vi "Read Camera Status 2.vi"(8 "error in (no error)":errorcluster, 11 "Interface in":refnum<class "Interface.lvclass">) -> (0 "error out":errorcluster, 2 "Camera Status":T1={"CUBE_EXPOSURE_TIME"=0.0, "CUBES_DONE"=1, "LAST_IMAGE_NAME"="", "DISK_SPACE"=0, "FRAMES_DONE"=0, "CCD_STATUS"="", "CURRENT_TEMPERATURE"=0, "TEMPERATURE_STATUS"="", "FRAME_EXPOSURE_TIME"=0, "CCD_POWER_STATUS"=FALSE, "SERIAL_NUMBER"=0, "ACQUIRING"=FALSE}, 3 "Interface out":refnum<class "Interface.lvclass">)   [LabVIEW 2018, in "Interface.lvclass"]
uses:
  Interface.lvclass
  Interface.lvclass/Interface.ctl
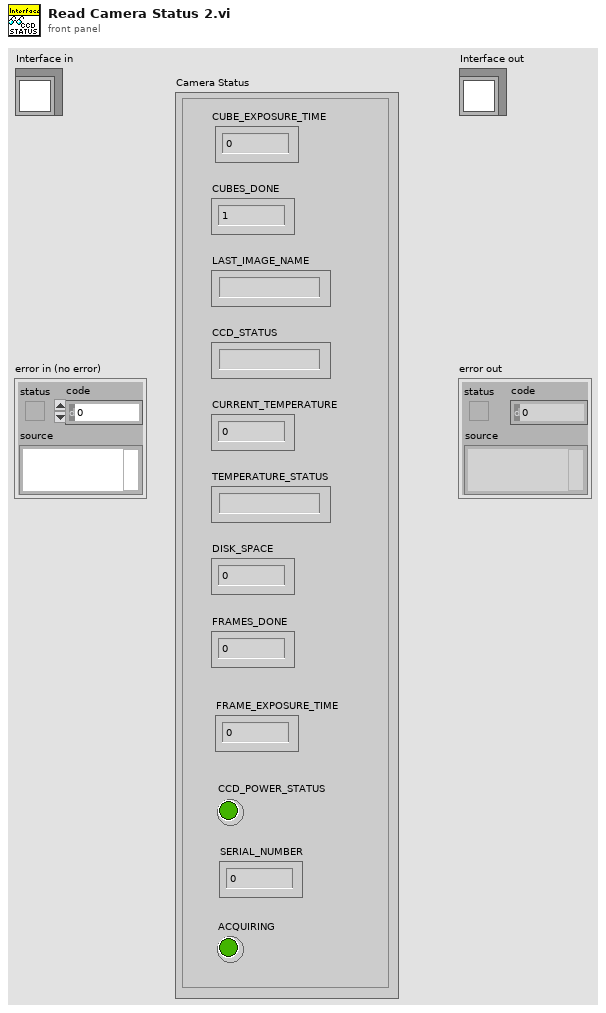
[diagram p1: front panel]
types:
  T1 = cluster{"CUBE_EXPOSURE_TIME":sgl, "CUBES_DONE":u16, "LAST_IMAGE_NAME":string, "DISK_SPACE":u16, "FRAMES_DONE":u16, "CCD_STATUS":string, "CURRENT_TEMPERATURE":i16, "TEMPERATURE_STATUS":string, "FRAME_EXPOSURE_TIME":u16, "CCD_POWER_STATUS":bool, "SERIAL_NUMBER":u16, "ACQUIRING":bool}
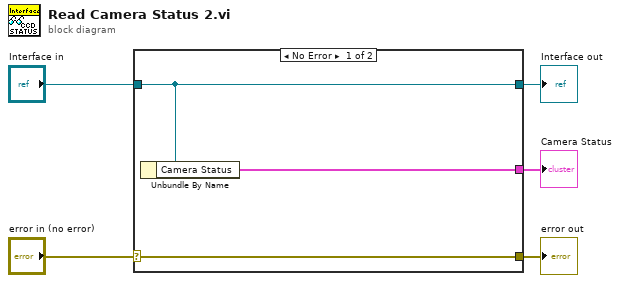
[diagram p0: block diagram]
diagram:
  n1 = case shown="No Error" "error in (no error)" {
    selector: "error in (no error)" -> [w8 w9]
    tunnel: [w8 w9] -> w4
    tunnel: [w7 w10] -> w2
    tunnel: "Interface in" -> [w7 w10]
    tunnel: [w6 _] -> w1
    frame No Error {
      n2 = Unbundle By Name(w7) -> ("Camera Status"=w6:T1)
    }
    frame Error {
    }
  }
  "error out" <- w4
  "Interface out" <- w2
  "Camera Status" <- w1
